vi "ADXRS453_Global.vi"() -> ()   [LabVIEW 2014]
panel:
  out "Gyro Angle":dbl
  out "Gyro Output (dps)":dbl
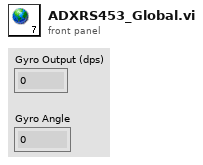
[diagram p1: front panel]
diagram:
